vi "Query Movement.vi"(8 "error in (no error)":errorcluster, 10 "Motor ID (0)":u8, 11 "Dynamixel Motor Simulator in":refnum<class "Dynamixel Motor Simulator.lvclass">) -> (0 "error out":errorcluster, 2 "Motor Moving":bool, 3 "Dynamixel Motor Simulator out":refnum<class "Dynamixel Motor Simulator.lvclass">)   [LabVIEW 2016, in "Dynamixel Motor Simulator.lvclass"]
doc: "Checks to see if the motor is attempting to reach its goal position."
uses:
  <instrlib>/Dynamixel Motor/HAIOL/Simulator/Dynamixel Motor Simulator.lvclass
  <instrlib>/Dynamixel Motor/HAIOL/Simulator/Dynamixel Motor Simulator.lvclass/Dynamixel Motor Simulator.ctl
  <vilib>/robotics/Simulator/Robot Factory/Motor/ODESimulator_Motor.lvclass
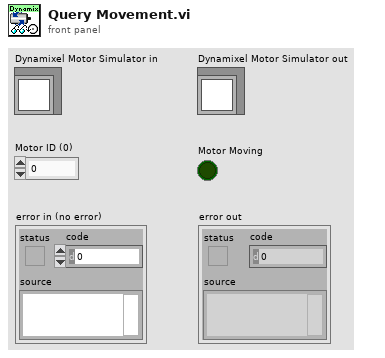
[diagram p1: front panel]
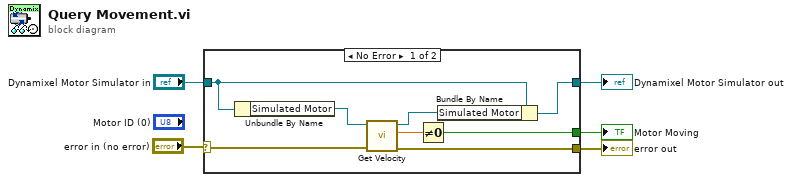
[diagram p0: block diagram]
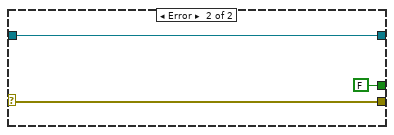
[diagram p2: hidden frame]
diagram:
  n1 = case shown="No Error" "error in (no error)" {
    selector: "error in (no error)" -> [w12 w15]
    tunnel: "Dynamixel Motor Simulator in" -> [w8 w16]
    tunnel: [w10 FALSE] -> w3
    tunnel: [w7 w16] -> w2
    tunnel: [w6 w15] -> w1
    frame No Error {
      n2 = Unbundle By Name(w8) -> ("Simulated Motor"=w13:refnum<class "ODESimulator_Motor.lvclass">)
      n3 = call-dynamic "Get Velocity.vi"("error in (no error)"=w12, "Motor in"=w13) -> ("error out"=w6:errorcluster, "CCW Velocity (rad/s)"=w11:dbl, "Motor out"=w9:refnum<class "ODESimulator_Motor.lvclass">)  [unwired: 7 in]
      n4 = Not Equal To 0?(x=w11) -> (x != 0?=w10:bool)
      n5 = Bundle By Name(cluster=w8, "Simulated Motor"=w9) -> (w7:refnum<class "Dynamixel Motor Simulator.lvclass">)
    }
    frame Error {
    }
  }
  "error out" <- w1
  "Dynamixel Motor Simulator out" <- w2
  "Motor Moving" <- w3
